vi "WriteIndicatorsToNT.vi"   [LabVIEW 2019]
uses:
  Globals/Sensor_Values.vi
  <vilib>/Rock Robotics/Network Tables/NT Write Number.vi
  <vilib>/Rock Robotics/Network Tables/NT Write Boolean.vi
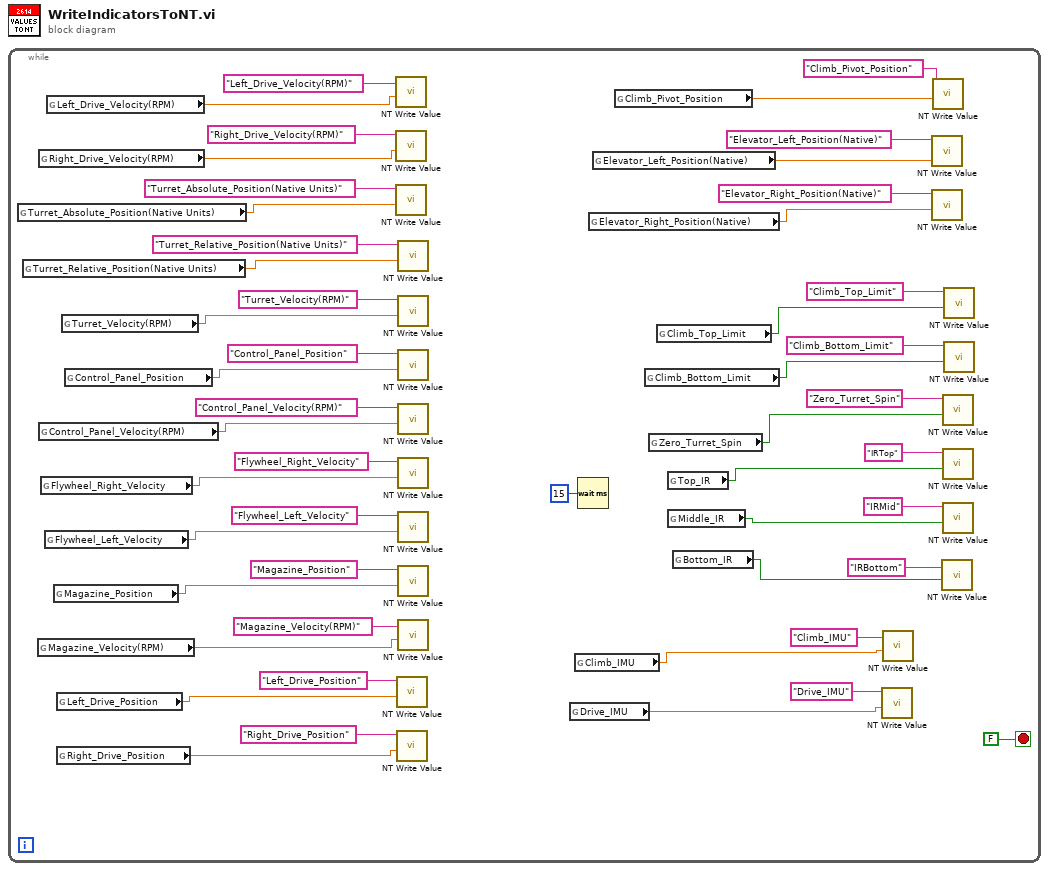
[diagram p0: block diagram]
diagram:
  n1 = while {
    stop <- FALSE stop-if-true
    n2 = global read "Sensor_Values.vi" "Turret_Absolute_Position(Native Units)"() -> (w9:dbl)
    n3 = global read "Sensor_Values.vi" "Turret_Relative_Position(Native Units)"() -> (w8:dbl)
    n4 = global read "Sensor_Values.vi" "Magazine_Velocity(RPM)"() -> (w39:dbl)
    n5 = global read "Sensor_Values.vi" "Right_Drive_Velocity(RPM)"() -> (w40:dbl)
    n6 = global read "Sensor_Values.vi" "Control_Panel_Velocity(RPM)"() -> (w35:dbl)
    n7 = global read "Sensor_Values.vi" "Flywheel_Right_Velocity"() -> (w36:dbl)
    n8 = global read "Sensor_Values.vi" "Flywheel_Left_Velocity"() -> (w37:dbl)
    n9 = global read "Sensor_Values.vi" "Left_Drive_Velocity(RPM)"() -> (w6:dbl)
    n10 = global read "Sensor_Values.vi" "Magazine_Position"() -> (w38:dbl)
    n11 = global read "Sensor_Values.vi" "Left_Drive_Position"() -> (w31:dbl)
    n12 = global read "Sensor_Values.vi" "Right_Drive_Position"() -> (w30:dbl)
    n13 = global read "Sensor_Values.vi" "Turret_Velocity(RPM)"() -> (w33:dbl)
    n14 = global read "Sensor_Values.vi" "Control_Panel_Position"() -> (w34:dbl)
    n15 = call-poly <vilib>:"NT Write Value.vi"("Numeric"=w6, "Name"="Left_Drive_Velocity(RPM)") -> ()  [unwired: 9 in, 1 out]
    n16 = call-poly <vilib>:"NT Write Value.vi"("Numeric"=w40, "Name"="Right_Drive_Velocity(RPM)") -> ()  [unwired: 9 in, 1 out]
    n17 = call-poly <vilib>:"NT Write Value.vi"("Numeric"=w9, "Name"="Turret_Absolute_Position(Native Units)") -> ()  [unwired: 9 in, 1 out]
    n18 = call-poly <vilib>:"NT Write Value.vi"("Numeric"=w31, "Name"="Left_Drive_Position") -> ()  [unwired: 9 in, 1 out]
    n19 = call-poly <vilib>:"NT Write Value.vi"("Numeric"=w30, "Name"="Right_Drive_Position") -> ()  [unwired: 9 in, 1 out]
    n20 = call-poly <vilib>:"NT Write Value.vi"("Numeric"=w8, "Name"="Turret_Relative_Position(Native Units)") -> ()  [unwired: 9 in, 1 out]
    n21 = call-poly <vilib>:"NT Write Value.vi"("Numeric"=w33, "Name"="Turret_Velocity(RPM)") -> ()  [unwired: 9 in, 1 out]
    n22 = call-poly <vilib>:"NT Write Value.vi"("Numeric"=w34, "Name"="Control_Panel_Position") -> ()  [unwired: 9 in, 1 out]
    n23 = call-poly <vilib>:"NT Write Value.vi"("Numeric"=w35, "Name"="Control_Panel_Velocity(RPM)") -> ()  [unwired: 9 in, 1 out]
    n24 = call-poly <vilib>:"NT Write Value.vi"("Numeric"=w36, "Name"="Flywheel_Right_Velocity") -> ()  [unwired: 9 in, 1 out]
    n25 = call-poly <vilib>:"NT Write Value.vi"("Numeric"=w37, "Name"="Flywheel_Left_Velocity") -> ()  [unwired: 9 in, 1 out]
    n26 = call-poly <vilib>:"NT Write Value.vi"("Numeric"=w38, "Name"="Magazine_Position") -> ()  [unwired: 9 in, 1 out]
    n27 = call-poly <vilib>:"NT Write Value.vi"("Numeric"=w39, "Name"="Magazine_Velocity(RPM)") -> ()  [unwired: 9 in, 1 out]
    n28 = global read "Sensor_Values.vi" "Drive_IMU"() -> (w1:dbl)
    n29 = global read "Sensor_Values.vi" "Climb_IMU"() -> (w2:dbl)
    n30 = Wait (ms)(milliseconds to wait=u32 15) -> ()  [unwired: 1 out]
    n31 = global read "Sensor_Values.vi" "Elevator_Right_Position(Native)"() -> (w14:dbl)
    n32 = global read "Sensor_Values.vi" "Elevator_Left_Position(Native)"() -> (w16:dbl)
    n33 = global read "Sensor_Values.vi" "Climb_Pivot_Position"() -> (w18:dbl)
    n34 = global read "Sensor_Values.vi" "Climb_Bottom_Limit"() -> (w10:bool)
    n35 = global read "Sensor_Values.vi" "Zero_Turret_Spin"() -> (w5:bool)
    n36 = global read "Sensor_Values.vi" "Climb_Top_Limit"() -> (w11:bool)
    n37 = global read "Sensor_Values.vi" "Top_IR"() -> (w28:bool)
    n38 = global read "Sensor_Values.vi" "Middle_IR"() -> (w27:bool)
    n39 = global read "Sensor_Values.vi" "Bottom_IR"() -> (w26:bool)
    n40 = call-poly <vilib>:"NT Write Value.vi"("Numeric"=w1, "Name"="Drive_IMU") -> ()  [unwired: 9 in, 1 out]
    n41 = call-poly <vilib>:"NT Write Value.vi"("Numeric"=w2, "Name"="Climb_IMU") -> ()  [unwired: 9 in, 1 out]
    n42 = call-poly <vilib>:"NT Write Value.vi"("Numeric"=w16, "Name"="Elevator_Left_Position(Native)") -> ()  [unwired: 9 in, 1 out]
    n43 = call-poly <vilib>:"NT Write Value.vi"("Numeric"=w14, "Name"="Elevator_Right_Position(Native)") -> ()  [unwired: 9 in, 1 out]
    n44 = call-poly <vilib>:"NT Write Value.vi"("Numeric"=w18, "Name"="Climb_Pivot_Position") -> ()  [unwired: 9 in, 1 out]
    n45 = call-poly <vilib>:"NT Write Value.vi"("Boolean"=w26, "Name"="IRBottom") -> ()  [unwired: 9 in, 1 out]
    n46 = call-poly <vilib>:"NT Write Value.vi"("Boolean"=w5, "Name"="Zero_Turret_Spin") -> ()  [unwired: 9 in, 1 out]
    n47 = call-poly <vilib>:"NT Write Value.vi"("Boolean"=w28, "Name"="IRTop") -> ()  [unwired: 9 in, 1 out]
    n48 = call-poly <vilib>:"NT Write Value.vi"("Boolean"=w27, "Name"="IRMid") -> ()  [unwired: 9 in, 1 out]
    n49 = call-poly <vilib>:"NT Write Value.vi"("Boolean"=w11, "Name"="Climb_Top_Limit") -> ()  [unwired: 9 in, 1 out]
    n50 = call-poly <vilib>:"NT Write Value.vi"("Boolean"=w10, "Name"="Climb_Bottom_Limit") -> ()  [unwired: 9 in, 1 out]
  }
